vi "main.vi"() -> ()   [LabVIEW 2023]
uses:
  cntrls/all_values.ctl
  cntrls/control_enum.ctl
panel:
  out "Counter 1":i32
  in  "Stop":bool
  out "VI2 Values":T1 {"Access counter value" format="%#_6f"; "SUM" format="%#_6f"; "Counter 2" format="%#_6f"}
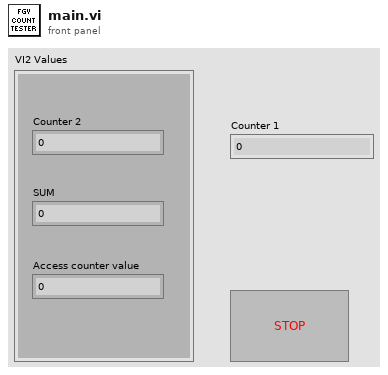
[diagram p1: front panel]
types:
  T1 = typedef "all_values.ctl" = cluster{"Counter 2":dbl, "SUM":dbl, "Access counter value":dbl}
  T2 = typedef "control_enum.ctl" = enum16{"read", "write", "clear"}
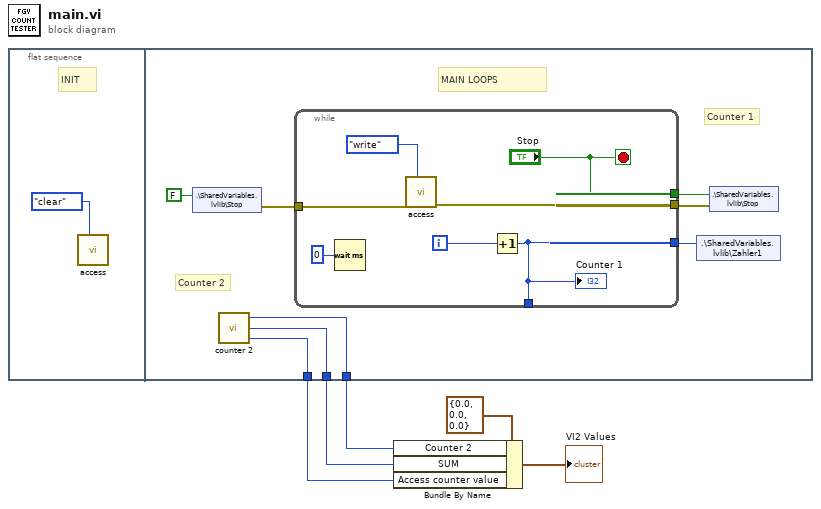
[diagram p0: block diagram]
diagram:
  n1 = flat-sequence {
    tunnel: [w12] -> w4
    tunnel: [w13] -> w3
    tunnel: [w14] -> w2
    frame #0 {
      # "INIT"
      n2 = call "access.vi"("Control_enum"=control_enum."clear") -> ()  [unwired: 7 in, 2 out]
    }
    frame #1 {
      # "Counter 2"
      # "Counter 1"
      # "MAIN LOOPS"
      n3 = shared-variable ".\\SharedVariables.lvlib\\Stop"(FALSE ("stop")) -> (error out=w7:errorcluster)  [unwired: 1 in]
      n4 = call "counter 2.vi"() -> ("Sum Counter 1+2"=w14:i32, "FGV value"=w13:u32, "Counter 2"=w12:i32)
      n5 = while {
        tunnel: [w19] -> w9
        tunnel: ["Stop"] -> w10
        tunnel: [w16] -> w11
        tunnel: [w16] -> _
        tunnel: w7 -> [w15]
        i -> [w18]
        stop <- "Stop" stop-if-true
        n6 = Wait (ms)(milliseconds to wait=u32 0) -> ()  [unwired: 1 out]
        n7 = call "access.vi"("Control_enum"=control_enum."write", "error in (no error)"=w15) -> ("error out"=w19:errorcluster)  [unwired: 6 in, 1 out]
        n8 = Increment(x=w18) -> (x+1=w16:i32)
        "Counter 1" <- w16
      }
      n9 = shared-variable ".\\SharedVariables.lvlib\\Zahler1"(w11) -> ()  [unwired: 1 in, 1 out]
      n10 = shared-variable ".\\SharedVariables.lvlib\\Stop"(w10, error in=w9) -> ()  [unwired: 1 out]
    }
  }
  n11 = Bundle By Name(cluster=T1 {"Counter 2"=0.0, "SUM"=0.0, "Access counter value"=0.0} ("ALL_VALUES 2"), "Counter 2"=w4, "SUM"=w3, "Access counter value"=w2) -> (→"VI2 Values":T1)
